vi "util.file.record.save.vi"(7 "delimiter (,)":string=":", 8 "error in":errorcluster, 9 "clk(NaN)":dbl=3814679003.515945, 10 "String Delimited Values":string="23.7:1464", 11 "record path in":string="OCS\\H1_TWET_2024-11-17.*") -> (0 "error out":errorcluster, 3 "Selected Folder":path=path "C:/interface/records/OCS/H1_TWET_2024-11-17.last")   [LabVIEW 2024]
doc: "Illustrates the various data types that the XY Graph accepts. Use the XY Graph to display data that is not uniformly distributed along the X-axis. This is particularly useful when displaying data that was sampled at a variable rate. The XY Graph is also useful for displaying data that is formatted as (X,Y) pairs."
uses:
  controls/typePathSelector.ctl
  <vilib>/Utility/error.llb/Clear Errors.vi
  <vilib>/Utility/file.llb/Write Delimited Spreadsheet (string).vi
  <vilib>/Utility/file.llb/Read Delimited Spreadsheet (DBL).vi
panel:
  out "appended array":string[](array[string])=["3814679003.52", "17/11/2024 11:03:23", "23.7", "1464", ""]
  out "date/time string":string="2024_07_03__filename.log"
  out "filename":string="03_07_2024"
  out "resulting string":string="03/07/2024_12:05:20"
  out "Multiple Plots (X Array and Y Array)":cluster{"all rows":dbl[], "all rows":dbl[]}[](graph)=[{"all rows"=[3802427858.71747, 3802427859.71747, 3802427861.71747, 3802427864.71747, 3802427868.71747, 3802427873.71747, 3802427879.71747, 3802427886.71747, 3802427894.71747, 3802427903.71747, 3802427913.71747, 3802427924.71747, 3802427936.71747, 3802427949.71747, 3802427963.71747, 3802427978.71747, 3802427994.71747, 3802428011.71747, 3802428029.71747, 3802428048.71747, 3802428068.71747, 3802428089.71747, 3802428111.71747, 3802428134.71747, 3802428158.71747, 3802428183.71747, 3802428209.71747, 3802428236.71747, 3802428264.71747, 3802428293.71747, 3802428323.71747, 3802428354.71747, 3802428386.71747, 3802428419.71747, 3802428453.71747, 3802428488.71747, 3802428524.71747, 3802428561.71747, 3802428599.71747, 3802428638.71747, 3802428678.71747, 3802428719.71747, 3802428761.71747, 3802428804.71747, 3802428848.71747, 3802428893.71747, 3802428939.71747, 3802428986.71747, 3802429034.71747, 3802429083.71747, 3802429133.71747, 3802429184.71747, 3802429236.71747, 3802429289.71747, 3802429343.71747, 3802429398.71747, 3802429454.71747, 3802429511.71747, 3802429569.71747, 3802429628.71747, 3802429688.71747, 3802429749.71747, 3802429811.71747, 3802429874.71747, 3802429938.71747, 3802430003.71747, 3802430069.71747, 3802430136.71747, 3802430204.71747, 3802430273.71747, 3802430343.71747, 3802430414.71747, 3802430486.71747, 3802430559.71747, 3802430633.71747, 3802430708.71747, 3802430784.71747, 3802430861.71747, 3802430939.71747, 3802431018.71747, 3802431098.71747, 3802431179.71747, 3802431261.71747, 3802431344.71747, 3802431428.71747, 3802431513.71747, 3802431599.71747, 3802431686.71747, 3802431774.71747, 3802431863.71747, 3802431953.71747, 3802432044.71747, 3802432136.71747, 3802432229.71747, 3802432323.71747, 3802432418.71747, 3802432514.71747, 3802432611.71747, 3802432709.71747, 3802432808.71747], "all rows"=[1.0, 0.998027, 0.992115, 0.982287, 0.968583, 0.951057, 0.929776, 0.904827, 0.876307, 0.844328, 0.809017, 0.770513, 0.728969, 0.684547, 0.637424, 0.587785, 0.535827, 0.481754, 0.425779, 0.368125, 0.309017, 0.24869, 0.187381, 0.125333, 0.062791, -0.0, -0.062791, -0.125333, -0.187381, -0.24869, -0.309017, -0.368125, -0.425779, -0.481754, -0.535827, -0.587785, -0.637424, -0.684547, -0.728969, -0.770513, -0.809017, -0.844328, -0.876307, -0.904827, -0.929776, -0.951057, -0.968583, -0.982287, -0.992115, -0.998027, -1.0, -0.998027, -0.992115, -0.982287, -0.968583, -0.951057, -0.929776, -0.904827, -0.876307, -0.844328, -0.809017, -0.770513, -0.728969, -0.684547, -0.637424, -0.587785, -0.535827, -0.481754, -0.425779, -0.368125, -0.309017, -0.24869, -0.187381, -0.125333, -0.062791, -0.0, 0.062791, 0.125333, 0.187381, 0.24869, 0.309017, 0.368125, 0.425779, 0.481754, 0.535827, 0.587785, 0.637424, 0.684547, 0.728969, 0.770513, 0.809017, 0.844328, 0.876307, 0.904827, 0.929776, 0.951057, 0.968583, 0.982287, 0.992115, 0.998027]}, {"all rows"=[3802427959.619741, 3802427960.619741, 3802427962.619741, 3802427965.619741, 3802427969.619741, 3802427974.619741, 3802427980.619741, 3802427987.619741, 3802427995.619741, 3802428004.619741, 3802428014.619741, 3802428025.619741, 3802428037.619741, 3802428050.619741, 3802428064.619741, 3802428079.619741, 3802428095.619741, 3802428112.619741, 3802428130.619741, 3802428149.619741, 3802428169.619741, 3802428190.619741, 3802428212.619741, 3802428235.619741, 3802428259.619741, 3802428284.619741, 3802428310.619741, 3802428337.619741, 3802428365.619741, 3802428394.619741, 3802428424.619741, 3802428455.619741, 3802428487.619741, 3802428520.619741, 3802428554.619741, 3802428589.619741, 3802428625.619741, 3802428662.619741, 3802428700.619741, 3802428739.619741, 3802428779.619741, 3802428820.619741, 3802428862.619741, 3802428905.619741, 3802428949.619741, 3802428994.619741, 3802429040.619741, 3802429087.619741, 3802429135.619741, 3802429184.619741, 3802429234.619741, 3802429285.619741, 3802429337.619741, 3802429390.619741, 3802429444.619741, 3802429499.619741, 3802429555.619741, 3802429612.619741, 3802429670.619741, 3802429729.619741, 3802429789.619741, 3802429850.619741, 3802429912.619741, 3802429975.619741, 3802430039.619741, 3802430104.619741, 3802430170.619741, 3802430237.619741, 3802430305.619741, 3802430374.619741, 3802430444.619741, 3802430515.619741, 3802430587.619741, 3802430660.619741, 3802430734.619741, 3802430809.619741, 3802430885.619741, 3802430962.619741, 3802431040.619741, 3802431119.619741, 3802431199.619741, 3802431280.619741, 3802431362.619741, 3802431445.619741, 3802431529.619741, 3802431614.619741, 3802431700.619741, 3802431787.619741, 3802431875.619741, 3802431964.619741, 3802432054.619741, 3802432145.619741, 3802432237.619741, 3802432330.619741, 3802432424.619741, 3802432519.619741, 3802432615.619741, 3802432712.619741, 3802432810.619741, 3802432909.619741], "all rows"=[0.0, 0.062791, 0.125333, 0.187381, 0.24869, 0.309017, 0.368125, 0.425779, 0.481754, 0.535827, 0.587785, 0.637424, 0.684547, 0.728969, 0.770513, 0.809017, 0.844328, 0.876307, 0.904827, 0.929776, 0.951057, 0.968583, 0.982287, 0.992115, 0.998027, 1.0, 0.998027, 0.992115, 0.982287, 0.968583, 0.951057, 0.929776, 0.904827, 0.876307, 0.844328, 0.809017, 0.770513, 0.728969, 0.684547, 0.637424, 0.587785, 0.535827, 0.481754, 0.425779, 0.368125, 0.309017, 0.24869, 0.187381, 0.125333, 0.062791, -0.0, -0.062791, -0.125333, -0.187381, -0.24869, -0.309017, -0.368125, -0.425779, -0.481754, -0.535827, -0.587785, -0.637424, -0.684547, -0.728969, -0.770513, -0.809017, -0.844328, -0.876307, -0.904827, -0.929776, -0.951057, -0.968583, -0.982287, -0.992115, -0.998027, -1.0, -0.998027, -0.992115, -0.982287, -0.968583, -0.951057, -0.929776, -0.904827, -0.876307, -0.844328, -0.809017, -0.770513, -0.728969, -0.684547, -0.637424, -0.587785, -0.535827, -0.481754, -0.425779, -0.368125, -0.309017, -0.24869, -0.187381, -0.125333, -0.062791]}]
  # "example: \nfolder1\\folder2\\filename.log"
  # "folder1\\folder2\\..\\folderN\\file.log"
  # "example:\nfolder1\\folder2\\filename.*"
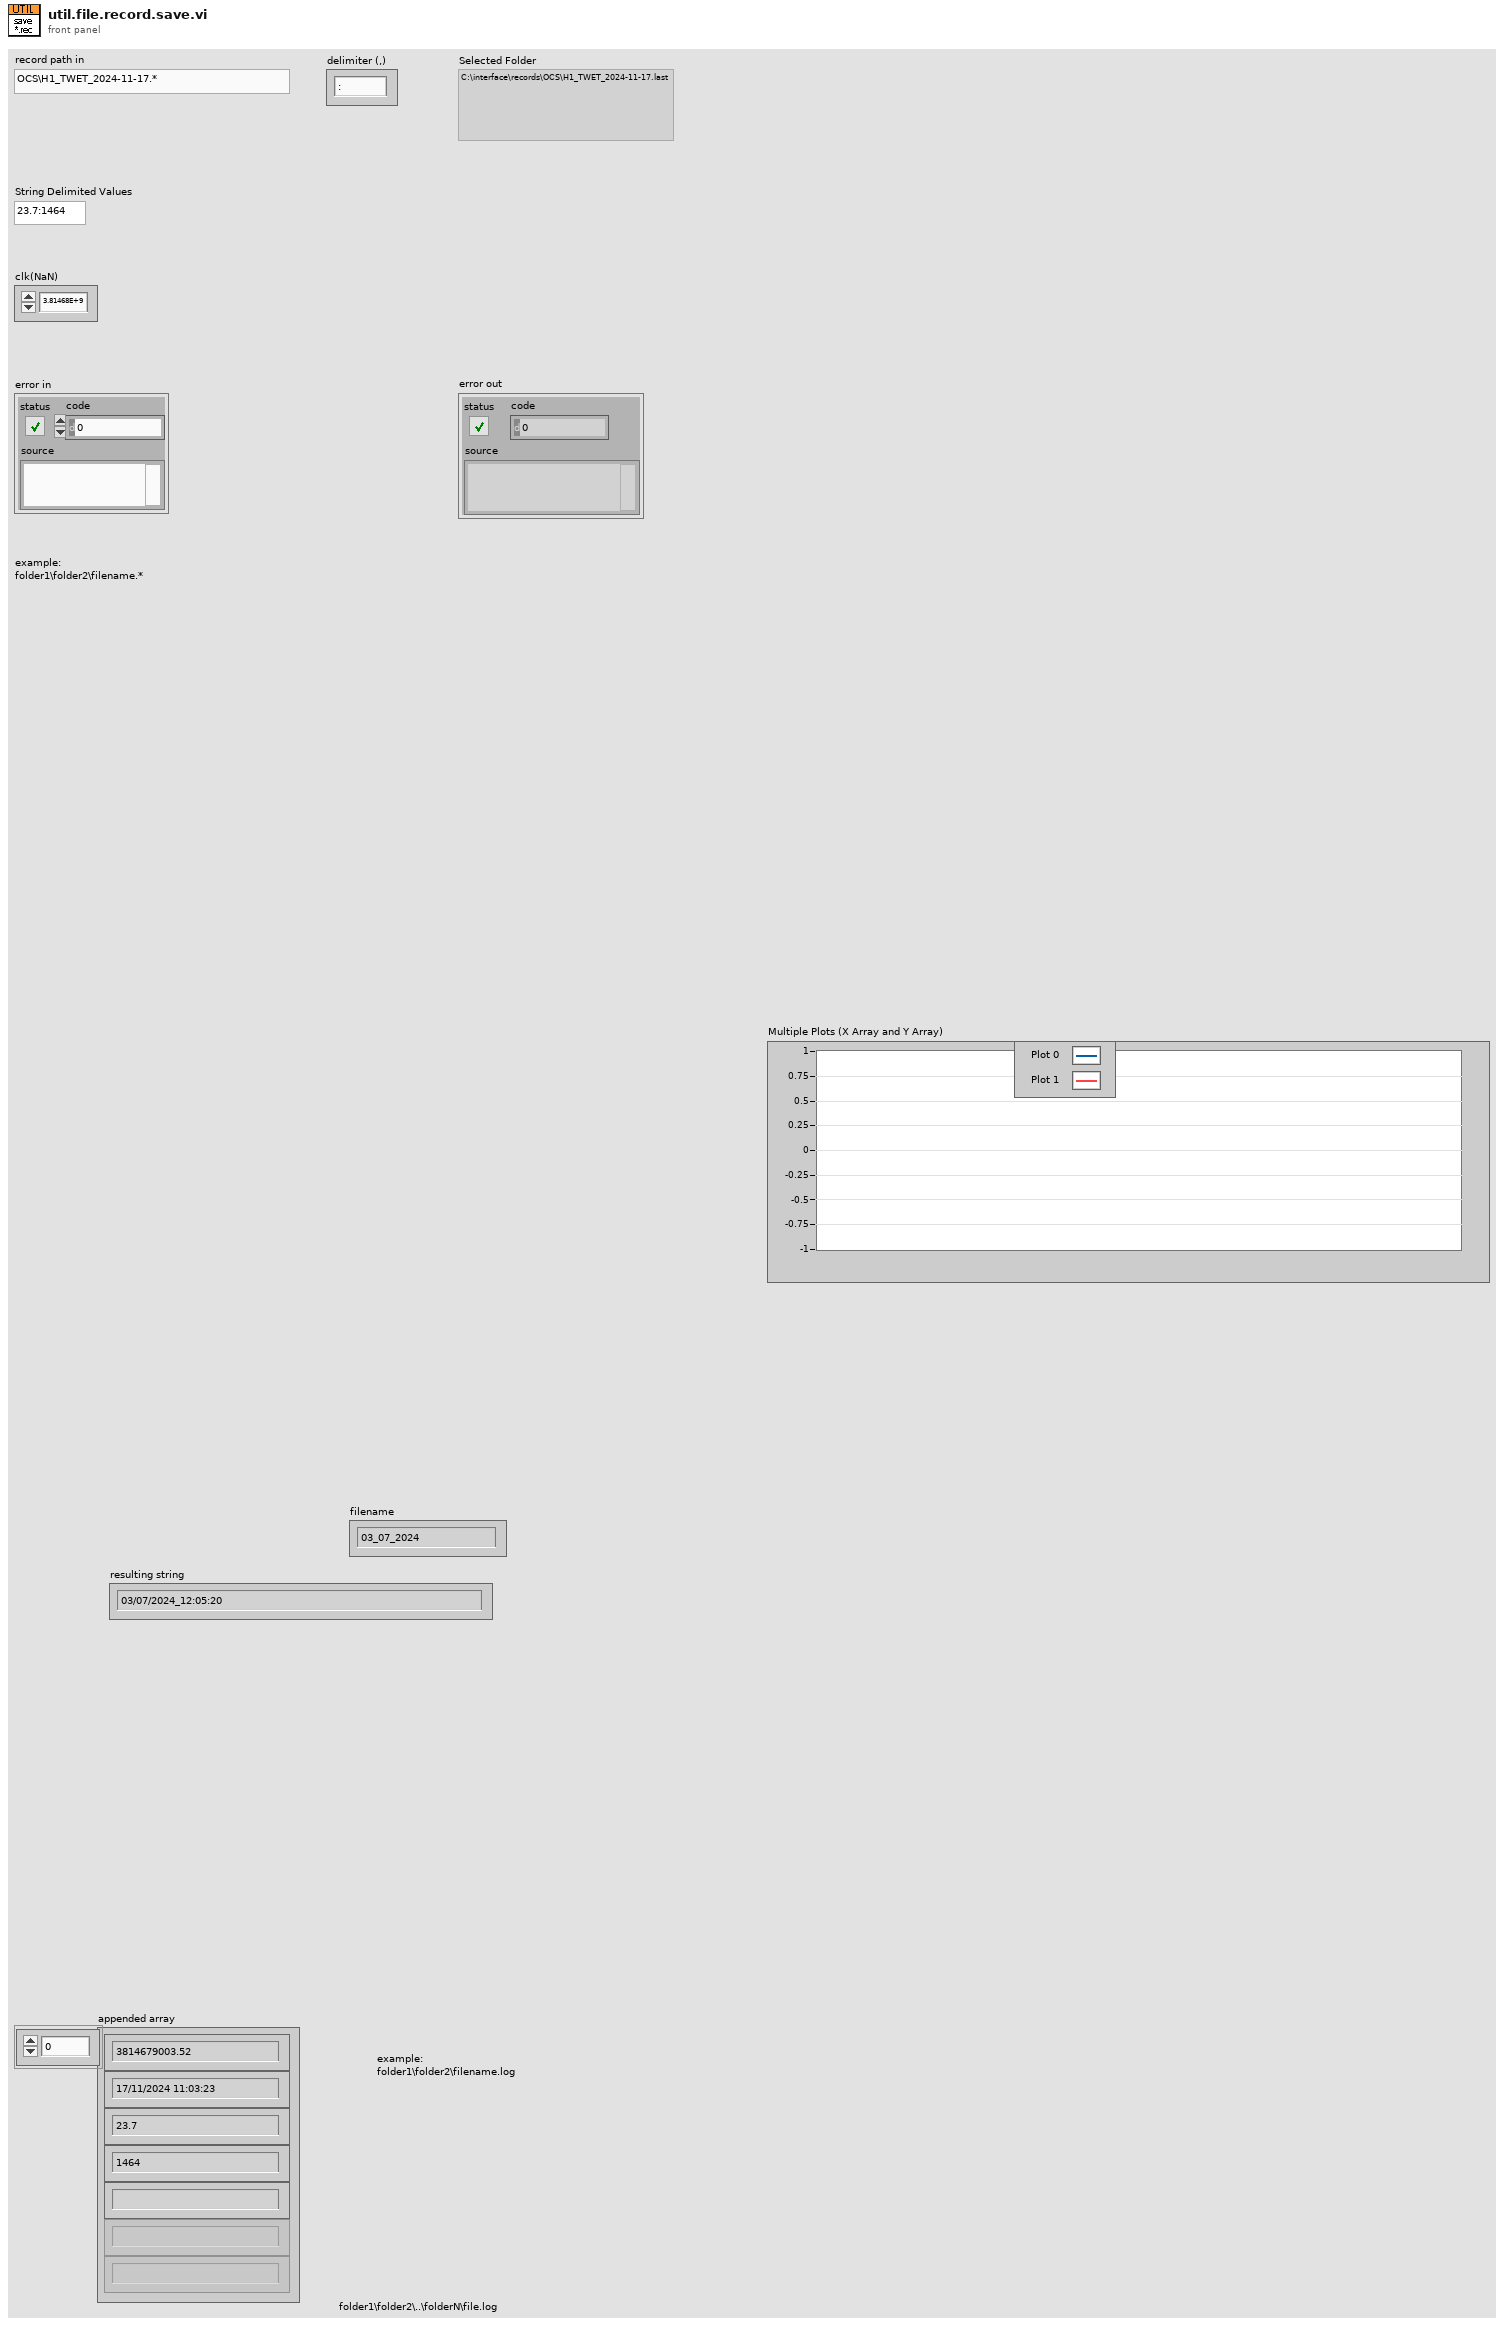
[diagram p1: front panel]
types:
  T1 = typedef "typePathSelector.ctl" = enum16{"DIR_PROCS", "DIR_CONFIG", "DIR_TEMPLATE", "DIR_IO_FILE", "DIR_RECORD", "DIR_LOG", "DIR_RUNTIME", "DIR_PRESET", "DIR_INI"}
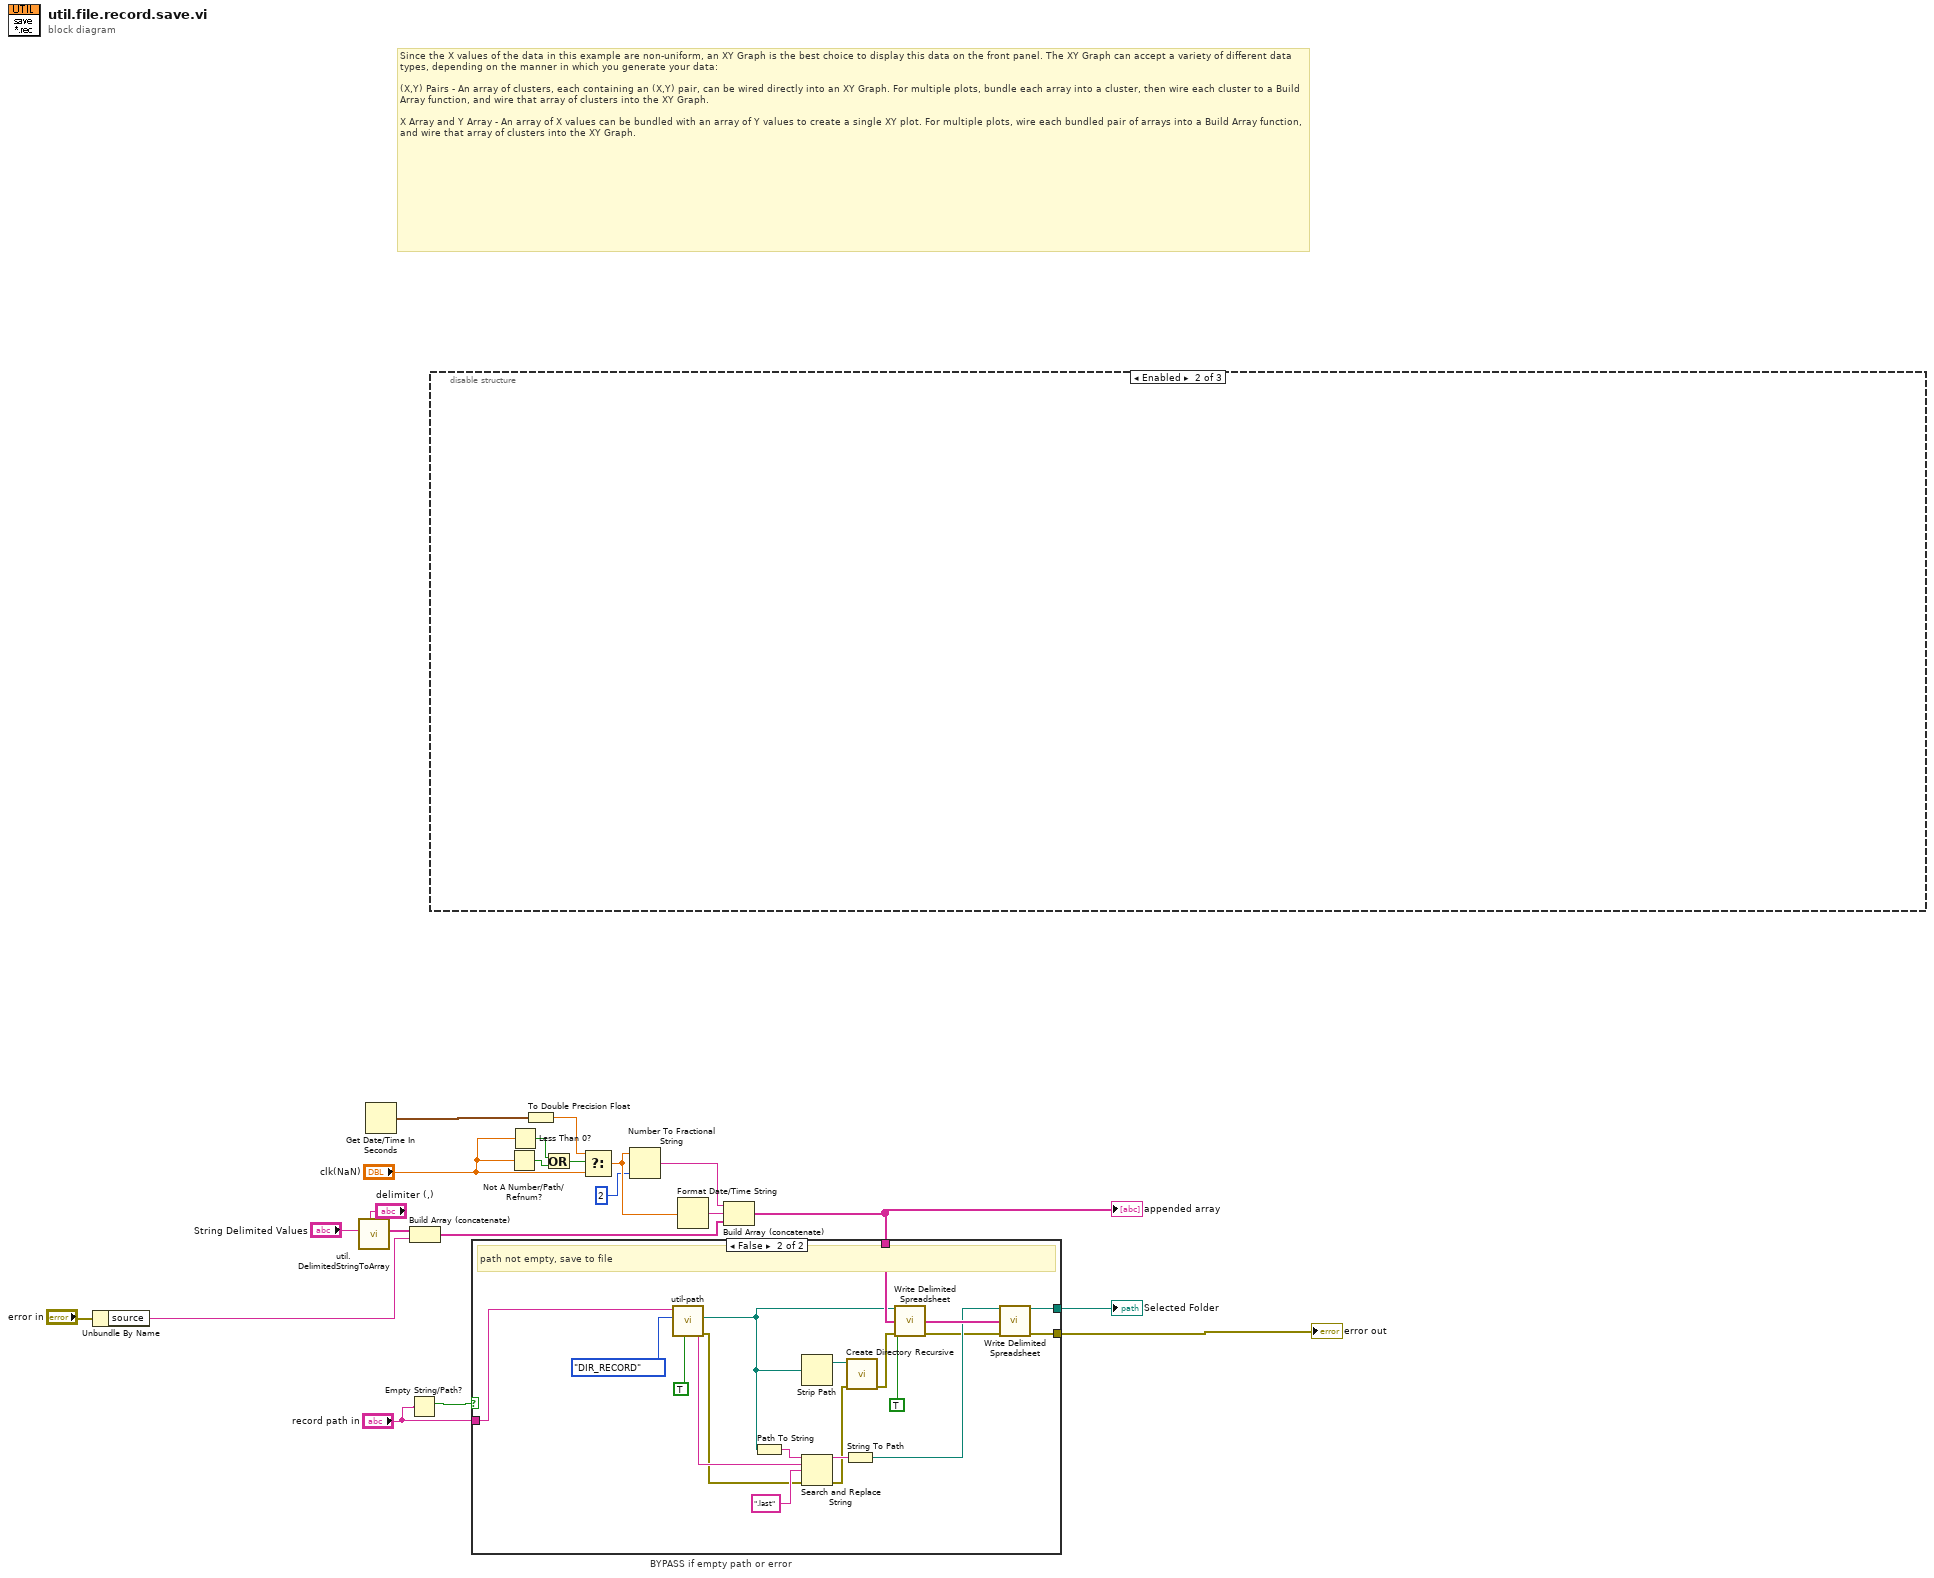
[diagram p0: block diagram]
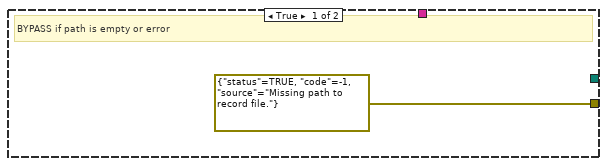
[diagram p2: hidden frame]
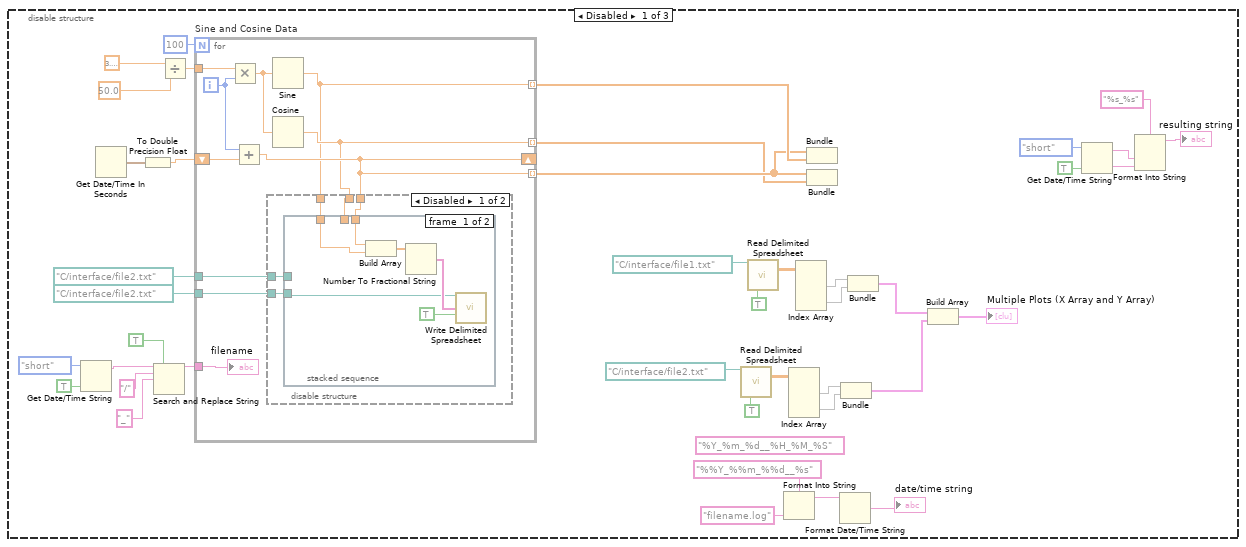
[diagram p3: hidden frame]
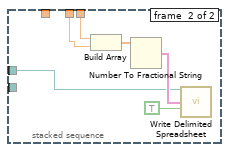
[diagram p4: hidden frame]
diagram:
  # "Since the X values of the data in this example are non-uniform, an XY Graph is the best choice to display this data on the front panel. The XY Graph can accept a variety of different data types, depending on the manner in which you generate your data:\n\n(X,Y) Pairs - An array of clusters, each containing an (X,Y) pair, can be wired directly into an XY Graph. For multiple plots, bundle each array into a cluster, then wire each cluster to a Build Array function, and wire that array of clusters into the XY Graph.\n\nX Array and Y Array - An array of X values can be bundled with an array of Y values to create a single XY plot. For multiple plots, wire each bundled pair of arrays into a Build Array function, and wire that array of clusters into the XY Graph."
  n1 = Unbundle By Name("error in") -> ("source"=w2:string)
  n2 = call "util.DelimitedStringToArray.vi"("delimiter (,)"="delimiter (,)", "delimitaed string"="String Delimited Values") -> ("array out"=w16:string[])  [unwired: 9 in]
  n3 = Get Date/Time In Seconds() -> (seconds since 1Jan1904=w13:timestamp)
  n4 = Empty String/Path?(string/path="record path in") -> (empty?=w5:bool)
  n5 = Build Array (concatenate)(w16, w2) -> (w1:string[])
  n6 = disable-structure shown="Enabled" {
    frame Disabled {
      (unwired) "%Y_%m_%d__%H_%M_%S" ("time format string (%c)")
      n7 = Get Date/Time String(date format (0)=enum16{"short", "long", "abbreviated"}."short", want seconds? (F)=TRUE) -> (date string=w39:string)  [unwired: 1 in, 1 out]
      n8 = Get Date/Time In Seconds() -> (seconds since 1Jan1904=w27:timestamp)
      n9 = To Double Precision Float(number=w27) -> (double precision float=w42:dbl)
      n10 = Search and Replace String(replace all?=TRUE ("replace all? (F)"), input string=w39, search string="/" ("input string"), replace string="_" ("input string")) -> (result string=w35:string)  [unwired: 4 in, 3 out]
      n11 = Divide(x=3.141592653589793, y=50.0) -> (x/y=w60:dbl)
      n12 = for "Sine and Cosine Data" {
        N: 100 -> [_]
        tunnel: w60 -> [w72]
        tunnel: [w63] -> w58 mode=indexing
        tunnel: [w67] -> w56 mode=indexing
        shift-right: [w68] -> _
        shift-left: w42 -> [w70]
        tunnel: [w68] -> w57 mode=indexing
        tunnel: w35 -> [w66]
        tunnel: path "C:/interface/file2.txt" ("file path (dialog if empty)") -> [w65]
        tunnel: path "C:/interface/file2.txt" ("file path (dialog if empty)") -> [w64]
        i -> [w69]
        n13 = Multiply(x=w72, y=w69) -> (x*y=w71:dbl)
        n14 = Add(x=w69, y=w70) -> (x+y=w68:dbl)
        n15 = Sine(x=w71) -> (sin(x)=w63:dbl)
        n16 = Cosine(x=w71) -> (cos(x)=w67:dbl)
        n17 = disable-structure shown="Disabled" {
          disable-tunnel: w68 -> [w77 _]
          disable-tunnel: w67 -> [w74 _]
          disable-tunnel: w65 -> [w73 _]
          disable-tunnel: w64 -> [w76 _]
          disable-tunnel: w63 -> [w75 _]
          frame Disabled {
            n18 = stacked-sequence {
              tunnel: w77 -> [w82 w88]
              tunnel: w76 -> [w79 _]
              tunnel: w75 -> [w78 _]
              tunnel: w74 -> [_ w85]
              tunnel: w73 -> [_ w84]
              frame #0 {
                n19 = Build Array(w82, w78) -> (w81:dbl[])
                n20 = Number To Fractional String(number=w81) -> (F-format string=w80:string[])  [unwired: 3 in]
                n21 = call-poly <vilib>:"Write Delimited Spreadsheet.vi"("file path (dialog if empty)"=w79, "1D data"=w80, "append to file? (new file:F)"=TRUE) -> ()  [unwired: 11 in, 2 out]
              }
              frame #1 {
                n22 = Build Array(w88, w85) -> (w87:dbl[])
                n23 = Number To Fractional String(number=w87) -> (F-format string=w86:string[])  [unwired: 3 in]
                n24 = call-poly <vilib>:"Write Delimited Spreadsheet.vi"("file path (dialog if empty)"=w84, "1D data"=w86, "append to file? (new file:F)"=TRUE) -> ()  [unwired: 11 in, 2 out]
              }
            }
          }
          frame Enabled {
          }
        }
        "filename" <- w66
      }
      n25 = call-poly <vilib>:"Read Delimited Spreadsheet.vi"("file path (dialog if empty)"=path "C:/interface/file2.txt", "transpose? (F)"=TRUE) -> ("all rows"=w45:dbl[][])  [unwired: 8 in, 5 out]
      n26 = call-poly <vilib>:"Read Delimited Spreadsheet.vi"("file path (dialog if empty)"=path "C:/interface/file1.txt", "transpose? (F)"=TRUE) -> ("all rows"=w53:dbl[][])  [unwired: 8 in, 5 out]
      n27 = Format Into String(format string="%%Y_%%m_%%d__%s" ("time format string (%c)"), "filename.log" ("input 1")) -> (resulting string=w25:string)  [unwired: 2 in, 1 out]
      n28 = Index Array(array=w45) -> (element #1=w47:dbl[], element #2=w48:dbl[])  [unwired: 4 in]
      n29 = Index Array(array=w53) -> (element #1=w51:dbl[], element #2=w50:dbl[])  [unwired: 4 in]
      n30 = Bundle(w57, w58) -> ()  [unwired: 1 in, 1 out]
      n31 = Bundle(w57, w56) -> ()  [unwired: 1 in, 1 out]
      n32 = Format Date/Time String(time format string (%c)=w25) -> (date/time string=→"date/time string":string)  [unwired: 2 in]
      n33 = Bundle("all rows"=w47, "all rows"=w48) -> (w43:cluster{"all rows":dbl[], "all rows":dbl[]})  [unwired: 1 in]
      n34 = Bundle("all rows"=w51, "all rows"=w50) -> (w49:cluster{"all rows":dbl[], "all rows":dbl[]})  [unwired: 1 in]
      n35 = Build Array(w49, w43) -> (→"Multiple Plots (X Array and Y Array)":cluster{"all rows":dbl[], "all rows":dbl[]}[])
      n36 = Get Date/Time String(date format (0)=enum16{"short", "long", "abbreviated"}."short", want seconds? (F)=TRUE) -> (date string=w32:string, time string=w31:string)  [unwired: 1 in]
      n37 = Format Into String(format string="%s_%s", w32, w31) -> (resulting string=→"resulting string":string)  [unwired: 2 in, 1 out]
    }
    frame Enabled {
    }
    frame Disabled {
    }
  }
  n38 = Not A Number/Path/Refnum?(number/path/refnum="clk(NaN)") -> (NaN/Path/Refnum?=w12:bool)
  n39 = Less Than 0?(x="clk(NaN)") -> (x < 0?=w10:bool)
  n40 = To Double Precision Float(number=w13) -> (double precision float=w8:dbl)
  n41 = Or(x=w10, y=w12) -> (x .or. y?=w11:bool)
  n42 = Select(t=w8, s=w11, f="clk(NaN)") -> (s? t:f=w7:dbl)
  n43 = Number To Fractional String(number=w7, precision (6)=i16 2) -> (F-format string=w6:string)  [unwired: 2 in]
  n44 = Format Date/Time String(seconds (now)=w7) -> (date/time string=w9:string)  [unwired: 2 in]
  n45 = Build Array (concatenate)(w6, w9, w1) -> (w19:string[])
  "appended array" <- w19
  n46 = case "BYPASS if empty path or error" shown="False" w5 {
    tunnel: w19 -> [_ w101]
    tunnel: [errorcluster {"status"=TRUE, "code"=-1, "source"="Missing path to record file."} ("error in") w102] -> w21
    tunnel: [_ w103] -> w18
    tunnel: "record path in" -> [_ w105]
    frame True {
      # "BYPASS if path is empty or error"
    }
    frame False {
      # "path not empty, save to file"
      n47 = call "util-path.vi"("Create Folders?(F)"=TRUE, "Selected Folder (PROCS)"=typePathSelector."DIR_RECORD" ("*Folder Select"), "append path (ie. folder\\filename.*)"=w105) -> ("error out"=w95:errorcluster, "SelectedPath"=w100:path, ".extension (.prc)"=w98:string)  [unwired: 4 in, 2 out]
      n48 = Path To String(path=w100) -> (string=w99:string)
      n49 = Strip Path(path=w100) -> (stripped path=w104:path)  [unwired: 1 out]
      n50 = Search and Replace String(input string=w99, search string=w98, replace string=".last" ("replace string (\"\")"), error in=w95) -> (result string=w96:string, error out=w93:errorcluster)  [unwired: 4 in, 2 out]
      n51 = String To Path(string=w96) -> (path=w94:path)
      n52 = call <vilib>:"Create Directory Recursive.vi"("error in (no error)"=w93, "directory"=w104) -> ("error out"=w106:errorcluster)  [unwired: 3 in, 2 out]
      n53 = call-poly <vilib>:"Write Delimited Spreadsheet.vi"("file path (dialog if empty)"=w100, "1D data"=w101, "append to file? (new file:F)"=TRUE, "error in (no error)"=w106) -> ("error out"=w92:errorcluster)  [unwired: 10 in, 1 out]
      n54 = call-poly <vilib>:"Write Delimited Spreadsheet.vi"("file path (dialog if empty)"=w94, "1D data"=w101, "error in (no error)"=w92) -> ("new file path (Not A Path if cancelled)"=w103:path, "error out"=w102:errorcluster)  [unwired: 11 in]
    }
  }
  "error out" <- w21
  "Selected Folder" <- w18
